vi "SetControlsVisibilityAndEnabledState.vi"(6 "error in (no error)":errorcluster, 8 "Enabled state (Enabled)":T2(ring), 9 "Visible (T)":bool=TRUE, 10 "Array":refnum<vi>[](array[refnum]), 11 "Control State Array":T1[](array[typedef])) -> (0 "error out":errorcluster, 3 "Control State Array (out)":T1[](array[typedef]))   [LabVIEW 2010]
doc: "Modifies state variable of the control indicated by the reference. States are: Visible (T/F), Enabled (Enabled, Disabled, Disabled and greyed out)"
uses:
  Types/ControlAttributes.ctl
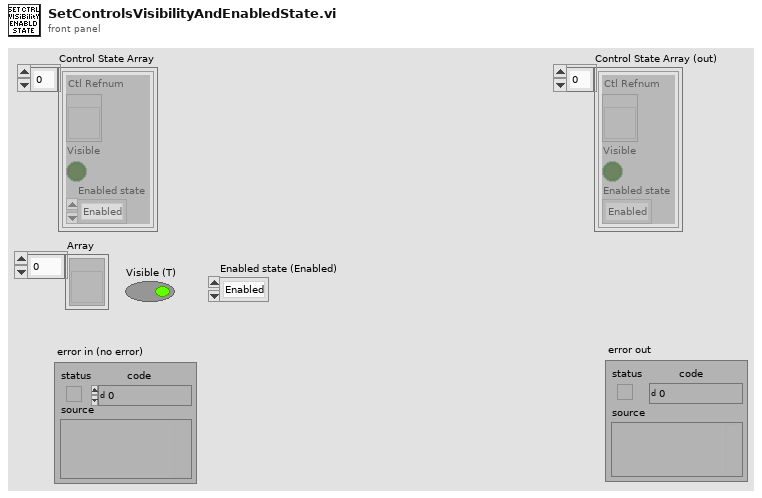
[diagram p1: front panel]
types:
  T1 = typedef "ControlAttributes.ctl" = cluster{"Ctl Refnum":refnum<vi>, "Visible":bool, "Enabled state":enum8{"Enabled", "Disabled", "Disabled and Grayed Out"}}
  T2 = enum8{"Enabled", "Disabled", "Disabled and Grayed Out"}
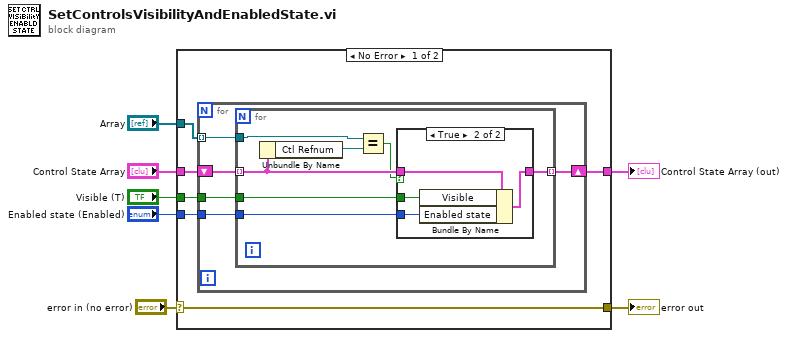
[diagram p0: block diagram]
diagram:
  n1 = case shown="No Error" "error in (no error)" {
    selector: "error in (no error)" -> [w13 w32]
    tunnel: [w13 w32] -> w6
    tunnel: "Control State Array" -> [w12 w31]
    tunnel: "Array" -> [w11 _]
    tunnel: "Enabled state (Enabled)" -> [w10 _]
    tunnel: "Visible (T)" -> [w9 _]
    tunnel: [w8 w31] -> w1
    frame No Error {
      n2 = for {
        tunnel: w11 -> [w18] mode=indexing
        tunnel: w10 -> [w15]
        tunnel: w9 -> [w16]
        shift-right: [w14] -> w8
        shift-left: w12 -> [w17]
        n3 = for {
          tunnel: w18 -> [w24]
          tunnel: w16 -> [w21]
          tunnel: w15 -> [w20]
          tunnel: w17 -> [w23] mode=indexing
          tunnel: [w22] -> w14 mode=indexing
          n4 = Unbundle By Name(w23) -> ("Ctl Refnum"=w25:refnum<vi>)
          n5 = Equal?(x=w24, y=w25) -> (x = y?=w19:bool)
          n6 = case shown="True" w19 {
            tunnel: w23 -> [w26 w30]
            tunnel: [w26 w29] -> w22
            tunnel: w21 -> [_ w28]
            tunnel: w20 -> [_ w27]
            frame False {
            }
            frame True {
              n7 = Bundle By Name(cluster=w30, "Visible"=w28, "Enabled state"=w27) -> (w29:T1)
            }
          }
        }
      }
    }
    frame Error {
    }
  }
  "error out" <- w6
  "Control State Array (out)" <- w1
